vi "TPIcontrol.vi"(8 "Fstep (kHz)":u32=5000, 9 "Freq (kHz)":u32=50000, 11 "Device index":u32=1) -> ()   [LabVIEW 2013]
panel:
  out "Write Buffer Freq":u8[](array[numeric])=[0, 85, 0, 2, 8, 1, 244] format="%x"
  out "Write Buffer":u8[](array[numeric])=[0, 85, 0, 2, 8, 1, 244] format="%x"
  out "Checksum":u8 format="%x"
  out "Checksum Step":u8 format="%x"
  out "Bytes Read Step":u32
  out "Read Buffer Step":u8[](array[numeric])=[0, 85, 0, 2, 8, 1, 244] format="%x"
  out "Checksum Freq":u8 format="%x"
  out "Bytes Read Freq":u32
  out "Read Buffer Freq":u8[](array[numeric])=[0, 85, 0, 2, 8, 1, 244] format="%x"
  out "Bytes Read":u32
  out "Read Buffer Out":u8[](array[numeric])=[0, 85, 0, 2, 8, 1, 244] format="%x"
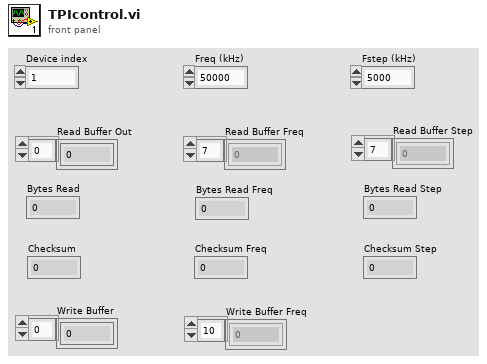
[diagram p1: front panel]
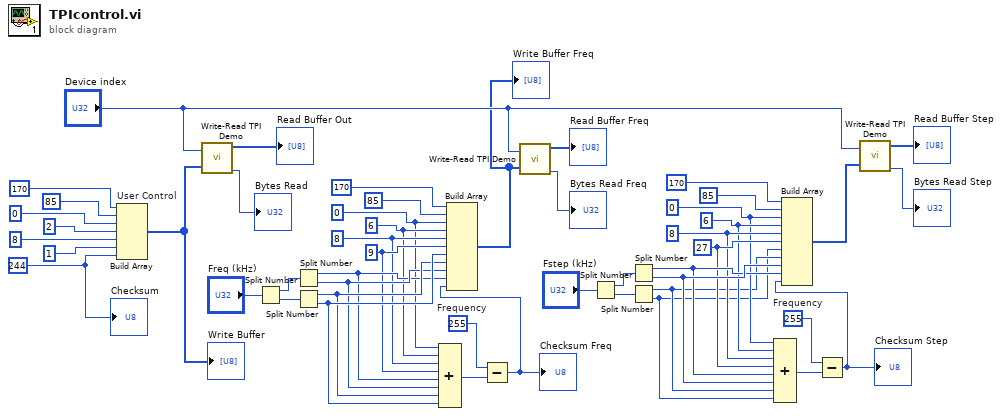
[diagram p0: block diagram]
diagram:
  w15 = u8 27
  w14 = u8 8
  w13 = u8 6
  w12 = u8 0
  w33 = u8 9
  w32 = u8 8
  w31 = u8 6
  w30 = u8 0
  w5 = u8 244
  n1 = Build Array "User Control"(u8 170, u8 85, u8 0, u8 2, u8 8, u8 1, w5) -> (w4:u8[])
  "Write Buffer" <- w4
  n2 = call "Write-Read TPI Demo.vi"("Write Buffer"=w4, "Device Index"="Device index") -> ("Bytes Read"=→"Bytes Read":u32, "Read Buffer Out"=→"Read Buffer Out":u8[])  [unwired: 2 in, 1 out]
  n3 = Split Number(x="Freq (kHz)") -> (hi(x)=w1:u16, lo(x)=w2:u16)
  n4 = Split Number(x=w1) -> (hi(x)=w34:u8, lo(x)=w35:u8)
  n5 = Split Number(x=w2) -> (hi(x)=w36:u8, lo(x)=w37:u8)
  n6 = Compound Arithmetic op=ADD(w30, w31, w32, w33, w34, w35, w36, w37) -> (w28:u8)
  n7 = Subtract(x=u8 255, y=w28) -> (x-y=w25:u8)
  "Checksum Freq" <- w25
  n8 = Build Array "Frequency"(u8 170, u8 85, w30, w31, w32, w33, w37, w36, w35, w34, w25) -> (w3:u8[])
  "Write Buffer Freq" <- w3
  n9 = call "Write-Read TPI Demo.vi"("Write Buffer"=w3, "Device Index"="Device index") -> ("Bytes Read"=→"Bytes Read Freq":u32, "Read Buffer Out"=→"Read Buffer Freq":u8[])  [unwired: 2 in, 1 out]
  n10 = Split Number(x="Fstep (kHz)") -> (hi(x)=w19:u16, lo(x)=w18:u16)
  n11 = Split Number(x=w19) -> (hi(x)=w16:u8, lo(x)=w17:u8)
  n12 = Split Number(x=w18) -> (hi(x)=w8:u8, lo(x)=w7:u8)
  n13 = Compound Arithmetic op=ADD(w12, w13, w14, w15, w16, w17, w8, w7) -> (w10:u8)
  n14 = Subtract(x=u8 255, y=w10) -> (x-y=w9:u8)
  "Checksum Step" <- w9
  n15 = Build Array "Frequency"(u8 170, u8 85, w12, w13, w14, w15, w7, w8, w17, w16, w9) -> (w6:u8[])
  n16 = call "Write-Read TPI Demo.vi"("Write Buffer"=w6, "Device Index"="Device index") -> ("Bytes Read"=→"Bytes Read Step":u32, "Read Buffer Out"=→"Read Buffer Step":u8[])  [unwired: 2 in, 1 out]
  "Checksum" <- w5
